vi "CompressAndUpdate(ScopeTrace).vi"(7 "force CVT update (false)":bool, 8 "error in":errorcluster, 9 "precision (12)":i16=12, 10 "Scope Trace":T1, 11 "command or variable name":string) -> (0 "error out":errorcluster, 3 "Trace String":string)   [LabVIEW 2011]
uses:
  trace_TypDef.ctl
  scopeTraceInfo_TypDEf.ctl
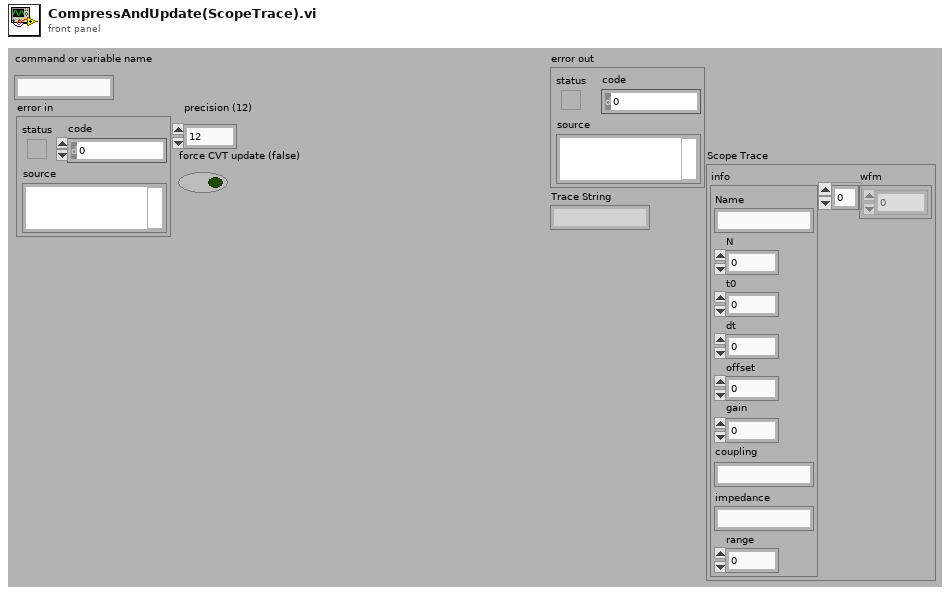
[diagram p1: front panel]
types:
  T1 = typedef "trace_TypDef.ctl" = cluster{"info":T2, "wfm":dbl[]}
  T2 = typedef "scopeTraceInfo_TypDEf.ctl" = cluster{"Name":string, "N":dbl, "t0":dbl, "dt":dbl, "offset":dbl, "gain":dbl, "coupling":string, "impedance":string, "range":dbl}
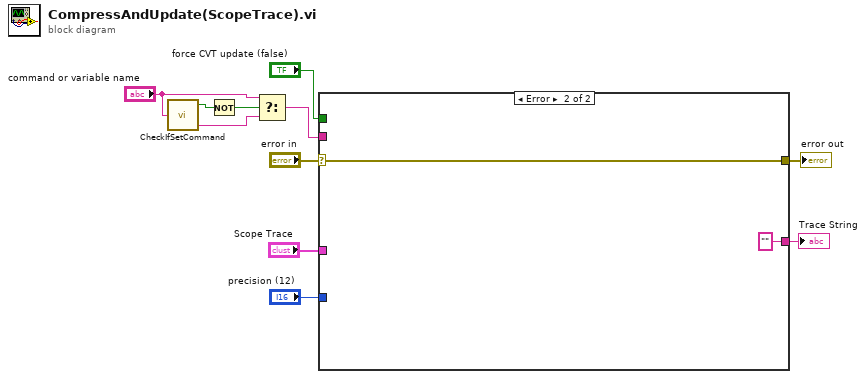
[diagram p0: block diagram]
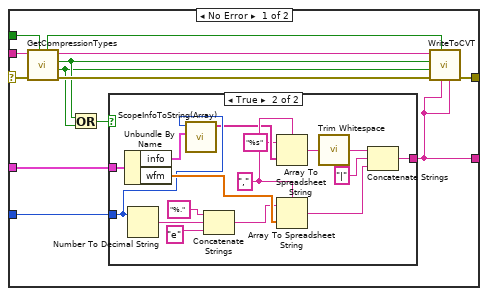
[diagram p2: hidden frame]
diagram:
  n1 = call "CheckIfSetCommand.vi"("Command"="command or variable name") -> ("setCommand?"=w8:bool, "variable"=w6:string)  [unwired: 1 out]
  n2 = Not(x=w8) -> (.not. x?=w9:bool)
  n3 = Select(t="command or variable name", s=w9, f=w6) -> (s? t:f=w5:string)
  n4 = case shown="Error" "error in" {
    selector: "error in" -> [w24 w42]
    tunnel: [w18 w42] -> w11
    tunnel: w5 -> [w19 _]
    tunnel: "Scope Trace" -> [w23 _]
    tunnel: "precision (12)" -> [w22 _]
    tunnel: "force CVT update (false)" -> [w17 _]
    tunnel: [w12 ""] -> w1
    frame No Error {
      n5 = call "GetCompressionTypes.vi"("force CVT update"=w17, "error in"=w24, "variable"=w19) -> ("error out"=w20:errorcluster, "non compressed"=w13:bool, "compressed"=w14:bool, "variable out"=w15:string, "force CVT update out"=w16:bool)  [unwired: 4 in]
      n6 = Or(x=w14, y=w13) -> (x .or. y?=w21:bool)
      n7 = case shown="True" w21 {
        tunnel: w23 -> [_ w37]
        tunnel: w22 -> [_ w27]
        tunnel: [_ w31] -> w12
        frame False {
        }
        frame True {
          w34 = "," ("delimiter (Tab)")
          n8 = Unbundle By Name(w37) -> ("info"=w28:T2, "wfm"=w36:dbl[])
          n9 = Number To Decimal String(number=w27) -> (decimal integer string=w39:string)  [unwired: 1 in]
          n10 = call "ScopeInfoToString(Array).vi"("info"=w28, "precision (12)"=w27) -> ("info string array"=w26:string[])  [unwired: 7 in, 2 out]
          n11 = Concatenate Strings("%." ("format string"), w39, "e" ("string")) -> (w35:string)
          n12 = Array To Spreadsheet String(delimiter (Tab)=w34, array=w26, 3:"%s" ("format string")) -> (spreadsheet string=w30:string)
          n13 = Array To Spreadsheet String(delimiter (Tab)=w34, array=w36, 3:w35) -> (spreadsheet string=w33:string)
          n14 = call "Trim Whitespace.vi"("string"=w30) -> ("trimmed string"=w29:string)  [unwired: 1 in]
          n15 = Concatenate Strings(w29, "|" ("string"), w33) -> (w31:string)
        }
      }
      n16 = call "WriteToCVT.vi"("non compressed string"=w12, "compressed string"=w12, "force CVT update"=w16, "error in"=w20, "non compressed"=w13, "compressed"=w14, "variable"=w15) -> ("error out"=w18:errorcluster)  [unwired: 4 in]
    }
    frame Error {
    }
  }
  "error out" <- w11
  "Trace String" <- w1
